vi "check_yw.vi"(8 "yw":string, 11 "lc_num":string) -> (0 "error":errorcluster caption="error out 4", 2 "check_yw":bool)   [LabVIEW 2017, in "Lib_code.lvlib"]
uses:
  Lib_code.lvlib
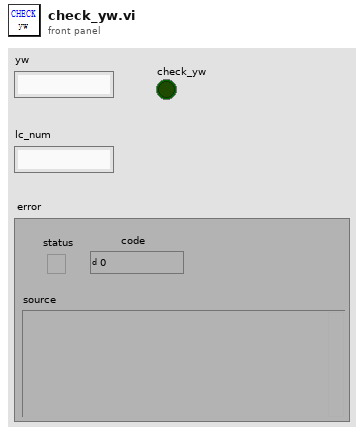
[diagram p1: front panel]
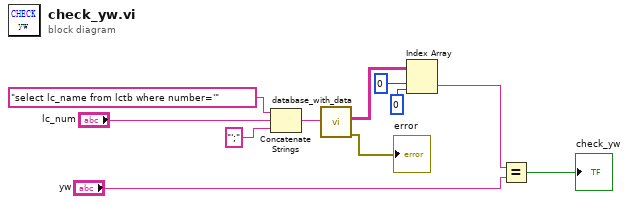
[diagram p0: block diagram]
diagram:
  n1 = Concatenate Strings("select lc_name from lctb where number='" ("字符串"), "lc_num", "';" ("字符串")) -> (w7:string)
  n2 = call "database_with_data.vi"("input"=w7) -> ("error"=→"error":errorcluster, "Data"=w1:string[][])  [unwired: 9 in]
  n3 = Index Array(array=w1, index (row)=0 ("索引 (行)"), index (col)=0 ("禁用的索引 (列)")) -> (element=w4:string)
  n4 = Equal?(x=w4, y="yw") -> (x = y?=→"check_yw":bool)
